vi "Create Linked List.vi"(10 "Letters (Default)":string[](array[string]), 11 "Text array to compress":string[](array[string])) -> (1 "Sorted Occurences":i32[](array[numeric]), 2 "Sorted Letters":string[](array[string]), 3 "Linked Nodes OUT":T1[](array[typedef]))   [LabVIEW 2017]
uses:
  BinaryNode.ctl
  <userlib>/_OpenG.lib/array/array.llb/Filter 1D Array with Scalar (String)__ogtk.vi
  <userlib>/_OpenG.lib/array/array.llb/Sort 1D Array (I32)__ogtk.vi
  <userlib>/_OpenG.lib/array/array.llb/Reorder 1D Array2 (String)__ogtk.vi
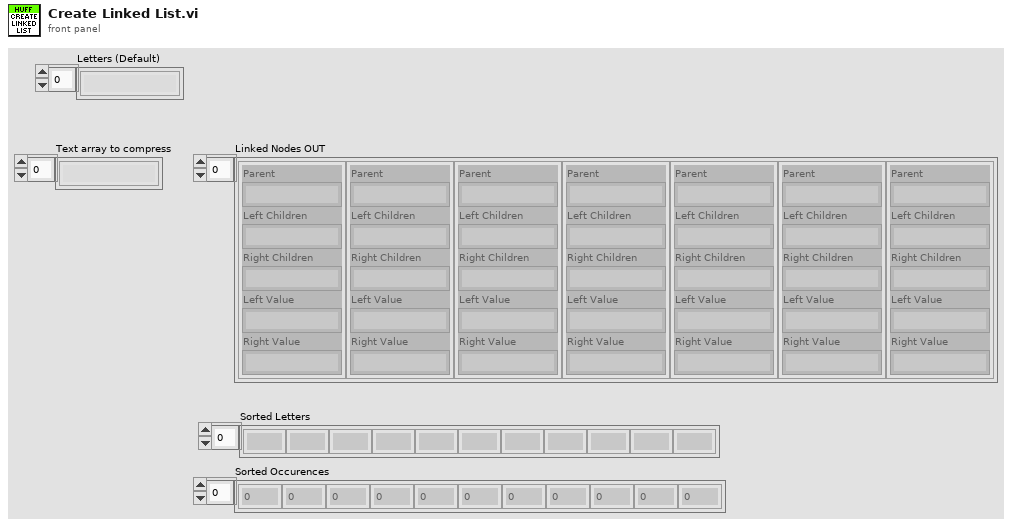
[diagram p1: front panel]
types:
  T1 = typedef "BinaryNode.ctl" = cluster{"Parent":string, "Left Children":string, "Right Children":string, "Left Value":string, "Right Value":string}
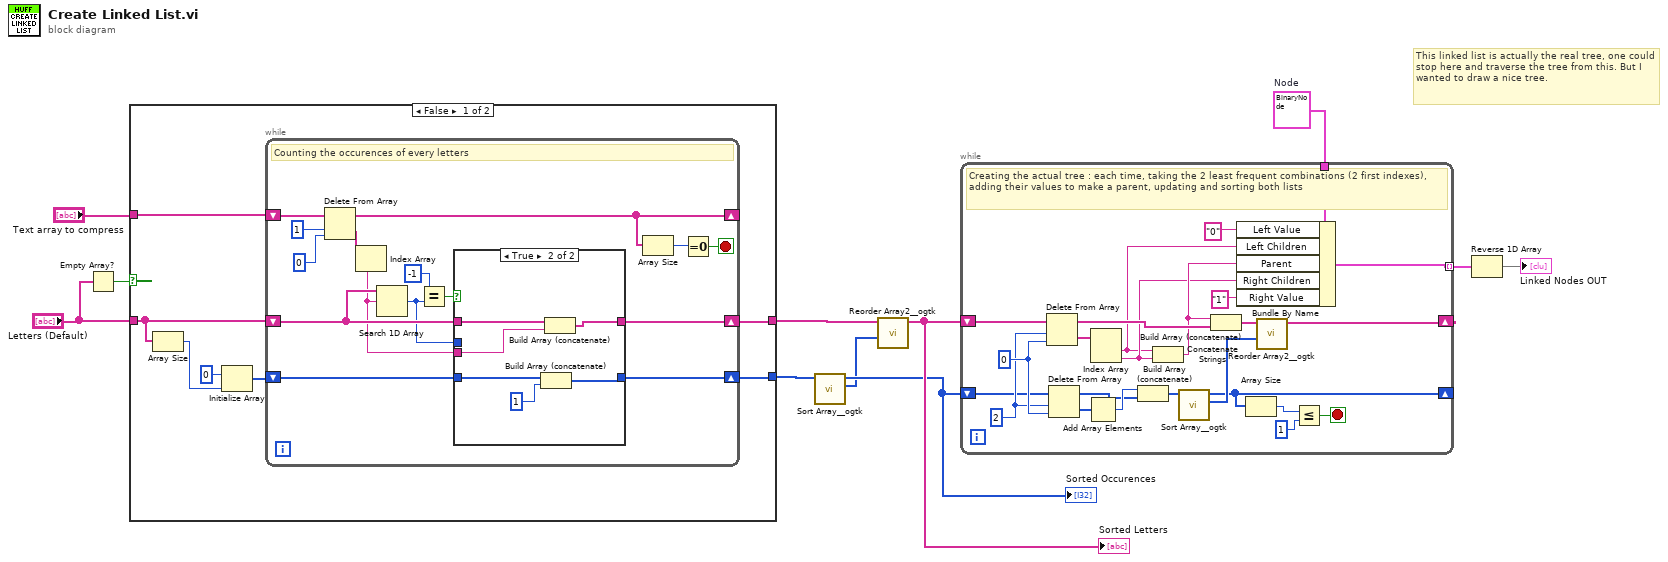
[diagram p0: block diagram]
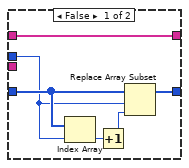
[diagram p2: hidden frame]
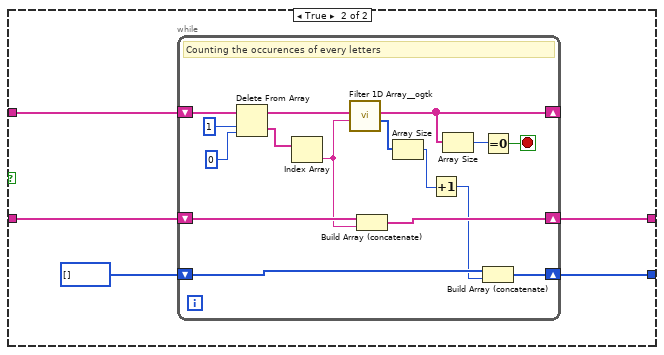
[diagram p3: hidden frame]
diagram:
  w9 = T1 {"Parent"="ROOT", "Left Children"="NULL", "Right Children"="NULL", "Left Value"="NULL", "Right Value"="NULL"}  # Node
  # "This linked list is actually the real tree, one could stop here and traverse the tree from this. But I wanted to draw a nice tree."
  n1 = Empty Array?(array="Letters (Default)") -> (empty?=w1:bool)
  n2 = case shown="False" w1 {
    tunnel: [w17 w50] -> w6
    tunnel: [w16 w49] -> w5
    tunnel: "Text array to compress" -> [w18 w48]
    tunnel: "Letters (Default)" -> [w15 w47]
    frame False {
      n3 = Array Size(array=w15) -> (size(s)=w14:i32)
      n4 = Initialize Array(0 ("element"), w14) -> (w13:i32[])
      n5 = while {
        shift-right: [w26] -> _
        shift-left: w18 -> [w29]
        shift-right: [w21] -> w17
        shift-left: w15 -> [w25]
        shift-right: [w22] -> w16
        shift-left: w13 -> [w23]
        stop <- w33 stop-if-true
        # "Counting the occurences of every letters"
        n6 = Delete From Array(array=w29, length=1 ("index"), index=0) -> (deleted portion=w28:string[], array with subset deleted=w26:string[])
        n7 = Index Array(array=w28) -> (element=w19:string)  [unwired: 1 in]
        n8 = Search 1D Array(1D array=w25, element=w19) -> (index of element=w20:i32)  [unwired: 1 in]
        n9 = Equal?(x=-1 ("index"), y=w20) -> (x = y?=w24:bool)
        n10 = case shown="True" w24 {
          tunnel: w25 -> [w39 w45]
          tunnel: w23 -> [w37 w42]
          tunnel: [w36 w40] -> w22
          tunnel: [w39 w43] -> w21
          tunnel: w20 -> [w35 _]
          tunnel: w19 -> [_ w44]
          frame False {
            n11 = Index Array(array=w37, index=w35) -> (element=w38:i32)
            n12 = Increment(x=w38) -> (x+1=w34:i32)
            n13 = Replace Array Subset(array=w37, new element=w34, index=w35) -> (w36:i32[])
          }
          frame True {
            n14 = Build Array (concatenate)(w42, 1 ("index")) -> (w40:i32[])
            n15 = Build Array (concatenate)(w45, w44) -> (w43:string[])
          }
        }
        n16 = Array Size(array=w26) -> (size(s)=w30:i32)
        n17 = Equal To 0?(x=w30) -> (x = 0?=w33:bool)
      }
    }
    frame True {
      n18 = while {
        shift-right: [w55] -> _
        shift-left: w48 -> [w58]
        shift-right: [w66] -> w50
        shift-left: w47 -> [w60]
        shift-right: [w64] -> w49
        shift-left: i32[] [] ("Occurences (Default)") -> [w65]
        stop <- w63 stop-if-true
        # "Counting the occurences of every letters"
        n19 = Delete From Array(array=w58, length=1 ("index"), index=0) -> (deleted portion=w51:string[], array with subset deleted=w56:string[])
        n20 = Index Array(array=w51) -> (element=w57:string)  [unwired: 1 in]
        n21 = call-poly <userlib>:"Filter 1D Array__ogtk.vi"("items to filter"=w57, "array"=w56) -> ("filtered item indices"=w53:i32[], "filtered array"=w55:string[])  [unwired: 4 in]
        n22 = Build Array (concatenate)(w60, w57) -> (w66:string[])
        n23 = Array Size(array=w53) -> (size(s)=w52:i32)
        n24 = Increment(x=w52) -> (x+1=w54:i32)
        n25 = Array Size(array=w55) -> (size(s)=w59:i32)
        n26 = Equal To 0?(x=w59) -> (x = 0?=w63:bool)
        n27 = Build Array (concatenate)(w65, w54) -> (w64:i32[])
      }
    }
  }
  n28 = call-poly <userlib>:"Sort Array__ogtk.vi"("Array in"=w5) -> ("Sorted Pointers"=w7:i32[], "Sorted Array out"=w8:i32[])  [unwired: 9 in]
  "Sorted Occurences" <- w8
  n29 = call-poly <userlib>:"Reorder Array2__ogtk.vi"("indices"=w7, "array"=w6) -> ("reordered array"=w11:string[])  [unwired: 9 in]
  "Sorted Letters" <- w11
  n30 = while {
    shift-right: [w76] -> _
    shift-left: w11 -> [w86]
    shift-right: [w77] -> _
    shift-left: w8 -> [w85]
    tunnel: w9 -> [w73]
    tunnel: [w67] -> w4 mode=indexing
    stop <- w78 stop-if-true
    w89 = 2
    w90 = 0
    # "Creating the actual tree : each time, taking the 2 least frequent combinations (2 first indexes), adding their values to make a parent, updating and sorting both lists"
    n31 = Delete From Array(array=w86, length=w89, index=w90) -> (deleted portion=w87:string[], array with subset deleted=w74:string[])
    n32 = Delete From Array(array=w85, length=w89, index=w90) -> (deleted portion=w88:i32[], array with subset deleted=w75:i32[])
    n33 = Add Array Elements(numeric array=w88) -> (sum=w84:i32)
    n34 = Index Array(array=w87) -> (element #1=w68:string, element #2=w70:string)  [unwired: 2 in]
    n35 = Build Array (concatenate)(w84, w75) -> (w82:i32[])
    n36 = Concatenate Strings(w68, w70) -> (w71:string)
    n37 = call-poly <userlib>:"Sort Array__ogtk.vi"("Array in"=w82) -> ("Sorted Pointers"=w83:i32[], "Sorted Array out"=w77:i32[])  [unwired: 9 in]
    n38 = Build Array (concatenate)(w71, w74) -> (w81:string[])
    n39 = Bundle By Name(cluster=w73, "Left Value"="0" ("Value"), "Left Children"=w68, "Parent"=w71, "Right Children"=w70, "Right Value"="1" ("Value")) -> (w67:T1)
    n40 = Array Size(array=w77) -> (size(s)=w80:i32)
    n41 = call-poly <userlib>:"Reorder Array2__ogtk.vi"("indices"=w83, "array"=w81) -> ("reordered array"=w76:string[])  [unwired: 9 in]
    n42 = Less Or Equal?(x=w80, y=1) -> (x <= y?=w78:bool)
  }
  n43 = Reverse 1D Array(array=w4) -> (reversed array=→"Linked Nodes OUT":T1[])
